vi "GetVertices.vi"(6 "error in":errorcluster, 9 "connection":T1) -> (0 "error out":errorcluster, 3 "connection out":T1, 4 "sink UID":i32, 5 "source UID":i32)   [LabVIEW 2014, in "Wire.lvclass"]
uses:
  Wire.lvclass
  ConnectionsTD.ctl
  Terminal/Terminal.lvclass
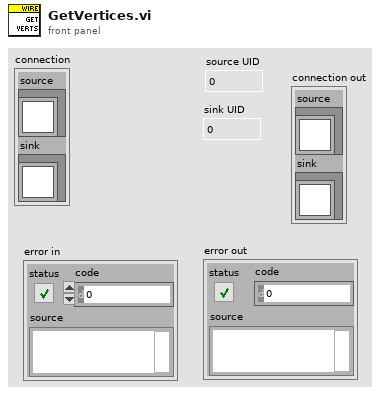
[diagram p1: front panel]
types:
  T1 = typedef "ConnectionsTD.ctl" = cluster{"source":refnum<class "Terminal.lvclass">, "sink":refnum<class "Terminal.lvclass">}
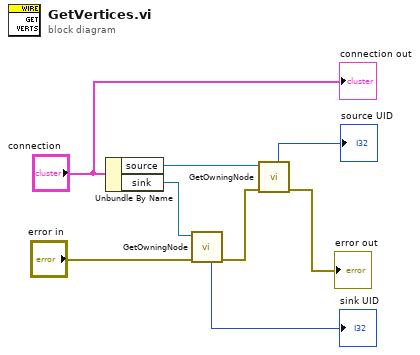
[diagram p0: block diagram]
diagram:
  n1 = Unbundle By Name("connection") -> ("source"=w8:refnum<class "Terminal.lvclass">, "sink"=w6:refnum<class "Terminal.lvclass">)
  n2 = call-dynamic "GetOwningNode.vi"("error in"="error in", "Terminal in"=w6) -> ("error out"=w4:errorcluster, "node UID"=→"sink UID":i32)  [unwired: 5 in, 1 out]
  n3 = call-dynamic "GetOwningNode.vi"("error in"=w4, "Terminal in"=w8) -> ("error out"=→"error out":errorcluster, "node UID"=→"source UID":i32)  [unwired: 5 in, 1 out]
  "connection out" <- "connection"
